vi "Init Max Size Data Array.vi"(10 "Data Stream Fmt Params":T2={"Samples per Block"=20, "Raw Data Status Len"=0, "Fltr Data Status Len"=0}, 11 "Data Collect Params":T1) -> (3 "initialized array":u32[][](array[numeric]))   [LabVIEW 2015, in "Collect Data Mgr.lvlib"]
uses:
  Collect Data Mgr.lvlib
  Tool Typedefs/_Data Stream Fmt Params Cluster--typedef.ctl
  Data Collect Parameters typedef--cluster.ctl
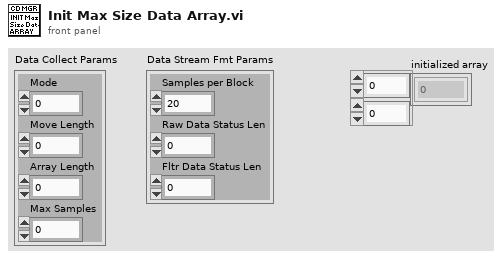
[diagram p1: front panel]
types:
  T1 = typedef "Collect Data Mgr.lvlib/Data Collect Parameters typedef--cluster.ctl" = cluster{"Mode":i8, "Move Length":i32, "Array Length":i32, "Max Samples":i32}
  T2 = typedef "_Data Stream Fmt Params Cluster--typedef.ctl" = cluster{"Samples per Block":i32, "Raw Data Status Len":i32, "Fltr Data Status Len":i32}
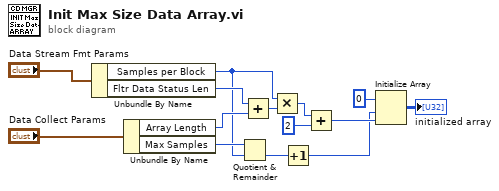
[diagram p0: block diagram]
diagram:
  n1 = Unbundle By Name("Data Stream Fmt Params") -> ("Samples per Block"=w3:i32, "Fltr Data Status Len"=w12:i32)
  n2 = Unbundle By Name("Data Collect Params") -> ("Array Length"=w11:i32, "Max Samples"=w13:i32)
  n3 = Quotient & Remainder(x=w13, y=w3) -> (floor(x/y)=w5:i32)  [unwired: 1 out]
  n4 = Add(x=w12, y=w11) -> (x+y=w10:i32)
  n5 = Multiply(x=w3, y=w10) -> (x*y=w9:i32)
  n6 = Increment(x=w5) -> (x+1=w4:i32)
  n7 = Add(x=w9, y=2) -> (x+y=w7:i32)
  n8 = Initialize Array(u32 0, w4, w7) -> (→"initialized array":u32[][])
